vi "Handle Refresh Response.vi"(6 "Refresh Token":string, 8 "error in (no error)":errorcluster, 10 "Response Body":string, 11 "Async Authorization in":refnum<class "Async Authorization.lvclass">) -> (0 "error out":errorcluster, 3 "Asyn Authorization out":refnum<class "Async Authorization.lvclass">)   [LabVIEW 2020, in "OAuth2.lvlib" / "Async Authorization.lvclass"]
uses:
  Async Authorization.lvclass
  Async Authorization.lvclass/Async Authorization.ctl
  Authorization/Authorization.lvclass
  50182fed-9479-4779-9116-d9088208cdec.vi
  3a5f6693-b230-4420-85c0-a79387339945.vi
  c54063c8-7f24-441d-9f2a-229ff977a01e.vi
  <vilib>/JDP Science/JSONtext/JSONtext.lvlib
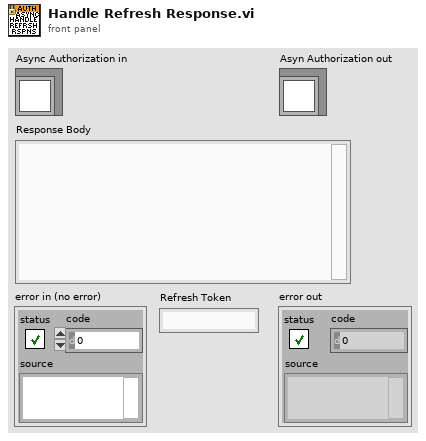
[diagram p1: front panel]
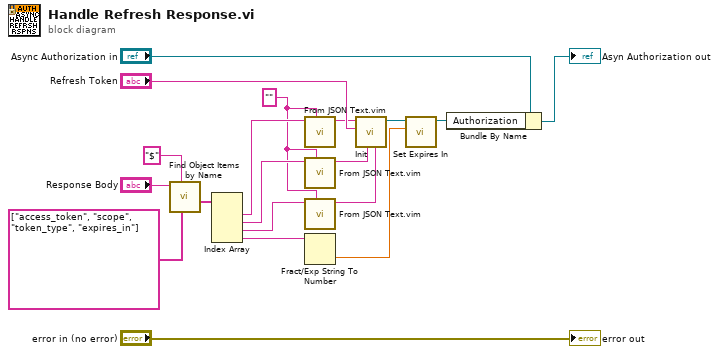
[diagram p0: block diagram]
diagram:
  w5 = ""
  n1 = call <vilib>:"Find Object Items by Name.vi"("Item Names"=string[] ["access_token", "scope", "token_type", "expires_in"] ("Search Keys"), "$Path or Item Name"="$", "JSON"="Response Body") -> ("<JSON>"=w1:string[])  [unwired: 6 in, 2 out]
  n2 = Index Array(array=w1) -> (element #1=w10:string, element #2=w8:string, element #3=w6:string, element #4=w18:string)  [unwired: 4 in]
  n3 = call "From JSON Text.vim"("Data Type and Default Value"=w5, "JSON"=w10) -> ("Data out"=w11:string)  [unwired: 8 in, 1 out]
  n4 = call "From JSON Text.vim"("Data Type and Default Value"=w5, "JSON"=w8) -> ("Data out"=w9:string)  [unwired: 8 in, 1 out]
  n5 = call "From JSON Text.vim"("Data Type and Default Value"=w5, "JSON"=w6) -> ("Data out"=w7:string)  [unwired: 8 in, 1 out]
  n6 = Fract/Exp String To Number(string=w18) -> (number=w16:dbl)  [unwired: 3 in, 1 out]
  n7 = call "Init.vi"("Token Type"=w7, "Scope"=w9, "Refresh Token"="Refresh Token", "Access Token"=w11) -> ("Authorization"=w17:refnum<class "Authorization.lvclass">)  [unwired: 7 in]
  n8 = call "Set Expires In.vi"("Expires In"=w16, "Authorization in"=w17) -> ("Authorization out"=w15:refnum<class "Authorization.lvclass">)  [unwired: 9 in]
  n9 = Bundle By Name(cluster="Async Authorization in", "Authorization"=w15) -> (→"Asyn Authorization out":refnum<class "Async Authorization.lvclass">)
  "error out" <- "error in (no error)"
